vi "Color Sensor V3 Color Match FGV.vi"(10 "FGV Cmd":T1, 11 "Color Match":T2) -> (3 "All Match Colors":T2[](array[typedef]))   [LabVIEW 2023]
uses:
  Typedef/Color Sensor V3 Color Match.ctl
  Typedef/Color Sensor V3 FGV Command.ctl
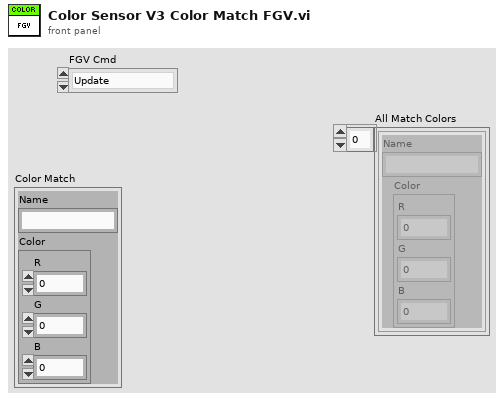
[diagram p1: front panel]
types:
  T1 = typedef "Color Sensor V3 FGV Command.ctl" = enum16{"Update", "Read"}
  T2 = typedef "Color Sensor V3 Color Match.ctl" = cluster{"Name":string, "Color":cluster{"R":dbl, "G":dbl, "B":dbl}}
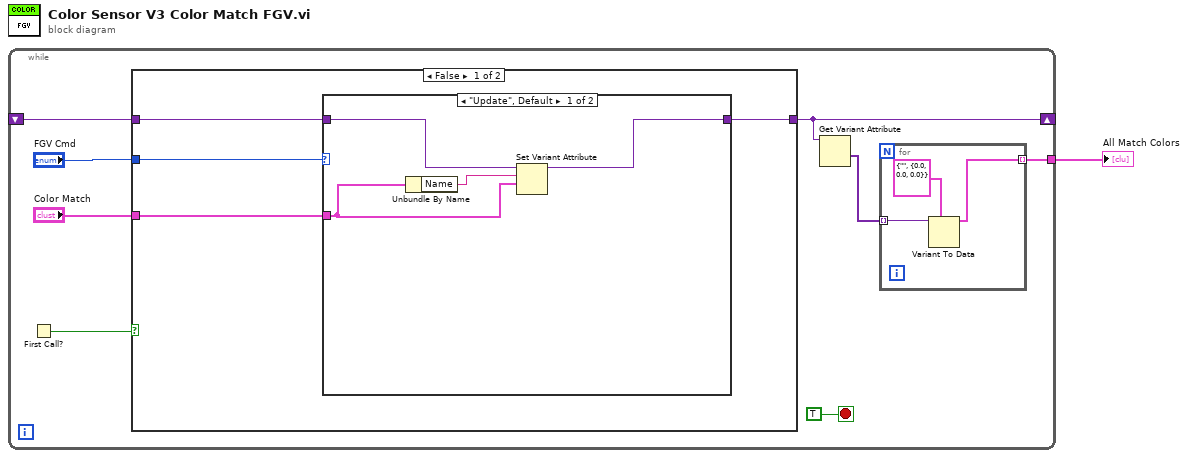
[diagram p0: block diagram]
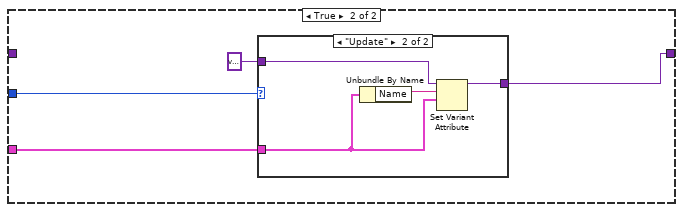
[diagram p3: hidden frame]
diagram:
  n1 = while {
    shift-right: [w5] -> _
    shift-left: _ -> [w7]
    tunnel: [w2] -> w1
    stop <- TRUE stop-if-true
    n2 = First Call?() -> (First Call?: T/F=w8:bool)
    n3 = case shown="False" w8 {
      tunnel: "Color Match" -> [w13 w23]
      tunnel: [w14 w24] -> w5
      tunnel: w7 -> [w15 _]
      tunnel: "FGV Cmd" -> [w16 w22]
      frame False {
        n4 = case shown="\"Update\", Default" w16 {
          tunnel: w15 -> [w20 w21]
          tunnel: [w19 w21] -> w14
          tunnel: w13 -> [w18 _]
          frame "Update", Default {
            n5 = Unbundle By Name(w18) -> ("Name"=w17:string)
            n6 = Set Variant Attribute(Variant=w20, name=w17, value=w18) -> (Variant out=w19:variant)  [unwired: 1 in, 2 out]
          }
          frame "Read" {
          }
        }
      }
      frame True {
        n7 = case shown="\"Update\"" w22 {
          tunnel: variant -> [w26 w30]
          tunnel: [w26 w29] -> w24
          tunnel: w23 -> [_ w28]
          frame Default {
          }
          frame "Update" {
            n8 = Unbundle By Name(w28) -> ("Name"=w27:string)
            n9 = Set Variant Attribute(Variant=w30, name=w27, value=w28) -> (Variant out=w29:variant)  [unwired: 1 in, 2 out]
          }
        }
      }
    }
    n10 = Get Variant Attribute(Variant=w5) -> (values=w4:variant[])  [unwired: 3 in, 3 out]
    n11 = for {
      tunnel: w4 -> [w12] mode=indexing
      tunnel: [w10] -> w2 mode=indexing
      n12 = Variant To Data(type=T2 {"Name"="", "Color"={"R"=0.0, "G"=0.0, "B"=0.0}} ("Color Match"), Variant=w12) -> (data=w10:T2)  [unwired: 1 in, 1 out]
    }
  }
  "All Match Colors" <- w1
